vi "Add Positon to Sidevi.vi"(8 "Direction":T1, 10 "Position":T3, 11 "Side Array":T2[](array[typedef])) -> (3 "Side Array Out":T2[](array[typedef]))   [LabVIEW 2024]
uses:
  Utility/Universal Utility/TypeDefs_Utility/Cluster_Row-Column.ctl
  Cluster_Side Datactl.ctl
  Utility/Universal Utility/TypeDefs_Utility/ENUM_4 Directions U-D-L-R.ctl
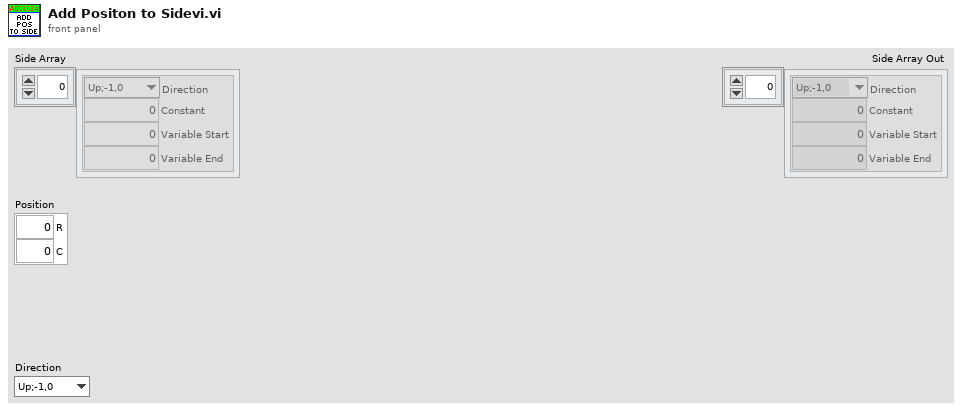
[diagram p1: front panel]
types:
  T1 = typedef "ENUM_4 Directions U-D-L-R.ctl" = enum16{"Up;-1,0", "Right;0,1", "Down;1,0", "Left;0,-1"}
  T2 = typedef "Cluster_Side Datactl.ctl" = cluster{"Direction":T1, "Constant":i32, "Variable Start":i32, "Variable End":i32}
  T3 = typedef "Cluster_Row-Column.ctl" = cluster{"R":i32, "C":i32}
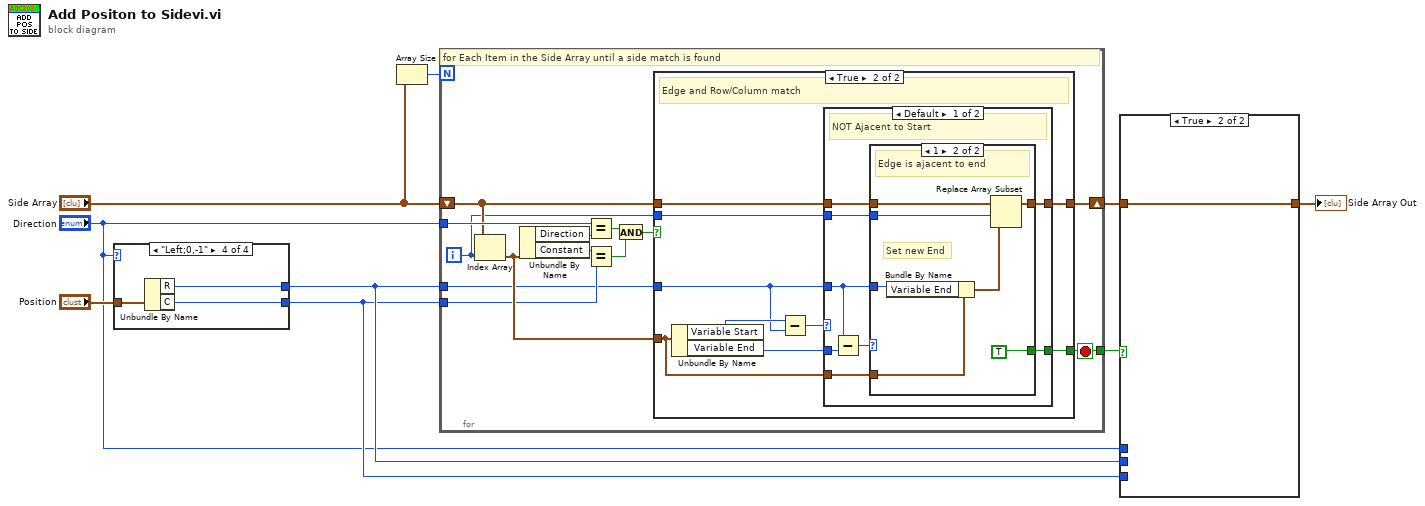
[diagram p0: block diagram]
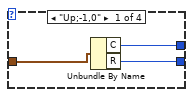
[diagram p2: hidden frame]
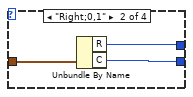
[diagram p3: hidden frame]
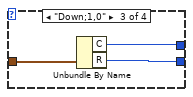
[diagram p4: hidden frame]
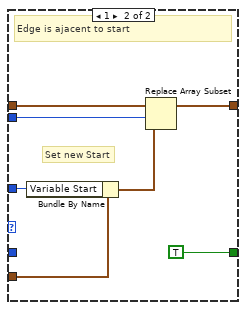
[diagram p7: hidden frame]
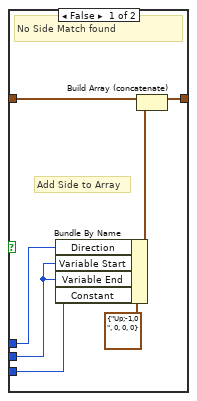
[diagram p8: hidden frame]
diagram:
  n1 = case shown="\"Left;0,-1\"" "Direction" {
    tunnel: "Position" -> [w12 w15 w18 w21]
    tunnel: [w11 w14 w17 w20] -> w4
    tunnel: [w10 w13 w16 w19] -> w5
    frame "Up;-1,0" {
      n2 = Unbundle By Name(w12) -> ("C"=w10:i32, "R"=w11:i32)
    }
    frame "Right;0,1" {
      n3 = Unbundle By Name(w15) -> ("R"=w13:i32, "C"=w14:i32)
    }
    frame "Down;1,0" {
      n4 = Unbundle By Name(w18) -> ("C"=w16:i32, "R"=w17:i32)
    }
    frame "Left;0,-1" {
      n5 = Unbundle By Name(w21) -> ("R"=w19:i32, "C"=w20:i32)
    }
  }
  n6 = Array Size(array="Side Array") -> (size(s)=w9:i32)
  n7 = for {
    N: w9 -> [_]
    tunnel: "Direction" -> [w33]
    shift-right: [w26] -> w8
    shift-left: "Side Array" -> [w28]
    tunnel: [w24] -> w7
    tunnel: w4 -> [w23]
    tunnel: w5 -> [w22]
    i -> [w25]
    stop <- w24 stop-if-true
    # "for Each Item in the Side Array until a side match is found"
    n8 = Index Array(array=w28, index=w25) -> (element=w27:T2)
    n9 = Unbundle By Name(w27) -> ("Direction"=w34:T1, "Constant"=w32:i32)
    n10 = Equal?(x=w33, y=w34) -> (x = y?=w30:bool)
    n11 = Equal?(x=w32, y=w23) -> (x = y?=w31:bool)
    n12 = And(x=w30, y=w31) -> (x .and. y?=w29:bool)
    n13 = case shown="True" w29 {
      tunnel: w28 -> [w35 w39]
      tunnel: w27 -> [_ w40]
      tunnel: [w35 w38] -> w26
      tunnel: w22 -> [_ w42]
      tunnel: w25 -> [_ w37]
      tunnel: [_ w36] -> w24
      frame False {
        # "No  match"
      }
      frame True {
        # "Edge and Row/Column match"
        n14 = Unbundle By Name(w40) -> ("Variable Start"=w43:i32, "Variable End"=w41:i32)
        n15 = Subtract(x=w43, y=w42) -> (x-y=w44:i32)
        n16 = case shown="Default" w44 {
          tunnel: w42 -> [w49 w63]
          tunnel: w41 -> [w52 _]
          tunnel: w40 -> [w50 w64]
          tunnel: w39 -> [w48 w67]
          tunnel: [w47 w66] -> w38
          tunnel: w37 -> [w46 w65]
          tunnel: [w45 TRUE] -> w36
          frame Default {
            # "NOT Ajacent to Start"
            n17 = Subtract(x=w49, y=w52) -> (x-y=w51:i32)
            n18 = case shown="1" w51 {
              tunnel: w50 -> [_ w60]
              tunnel: w49 -> [_ w59]
              tunnel: w48 -> [w53 w58]
              tunnel: [w53 w57] -> w47
              tunnel: w46 -> [_ w56]
              tunnel: [_ TRUE] -> w45
              frame Default {
                # "NOT ajacent to end"
              }
              frame 1 {
                # "Set new End"
                # "Edge is ajacent to end"
                n19 = Bundle By Name(cluster=w60, "Variable End"=w59) -> (w55:T2)
                n20 = Replace Array Subset(array=w58, new element=w55, index=w56) -> (w57:T2[])
              }
            }
          }
          frame 1 {
            # "Set new Start"
            # "Edge is ajacent to start"
            n21 = Bundle By Name(cluster=w64, "Variable Start"=w63) -> (w62:T2)
            n22 = Replace Array Subset(array=w67, new element=w62, index=w65) -> (w66:T2[])
          }
        }
      }
    }
  }
  n23 = case shown="True" w7 {
    tunnel: w8 -> [w74 w75]
    tunnel: [w73 w75] -> w2
    tunnel: w5 -> [w70 _]
    tunnel: w4 -> [w68 _]
    tunnel: "Direction" -> [w71 _]
    frame False {
      # "Add Side to Array"
      # "No Side Match found"
      n24 = Bundle By Name(cluster=T2 {"Direction"=enum."Up;-1,0", "Constant"=0, "Variable Start"=0, "Variable End"=0} ("element"), "Direction"=w71, "Variable Start"=w70, "Variable End"=w70, "Constant"=w68) -> (w69:T2)
      n25 = Build Array (concatenate)(w74, w69) -> (w73:T2[])
    }
    frame True {
    }
  }
  "Side Array Out" <- w2
